vi "HMU Cal - Get Optimal TX IF Frequency.vi"(5 "RF Frequency (Hz)":dbl format="%#_6p", 11 "error in (no error)":errorcluster) -> (6 "IF Frequency (Hz)":dbl format="%#_6p", 15 "error out":errorcluster)   [LabVIEW 2023, in "RFFixtureCharact.RFPM.lvlib" / "SG SC2250 Path.lvclass"]
uses:
  SG SC2250 Path.lvclass
  <vilib>/Utility/error.llb/Error Cluster From Error Code.vi
  <vilib>/ErrorRing/Error Ring.xnode
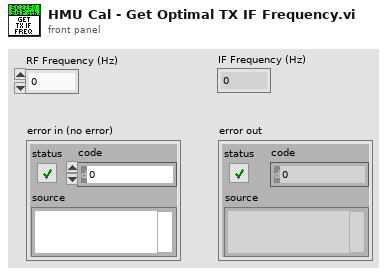
[diagram p1: front panel]
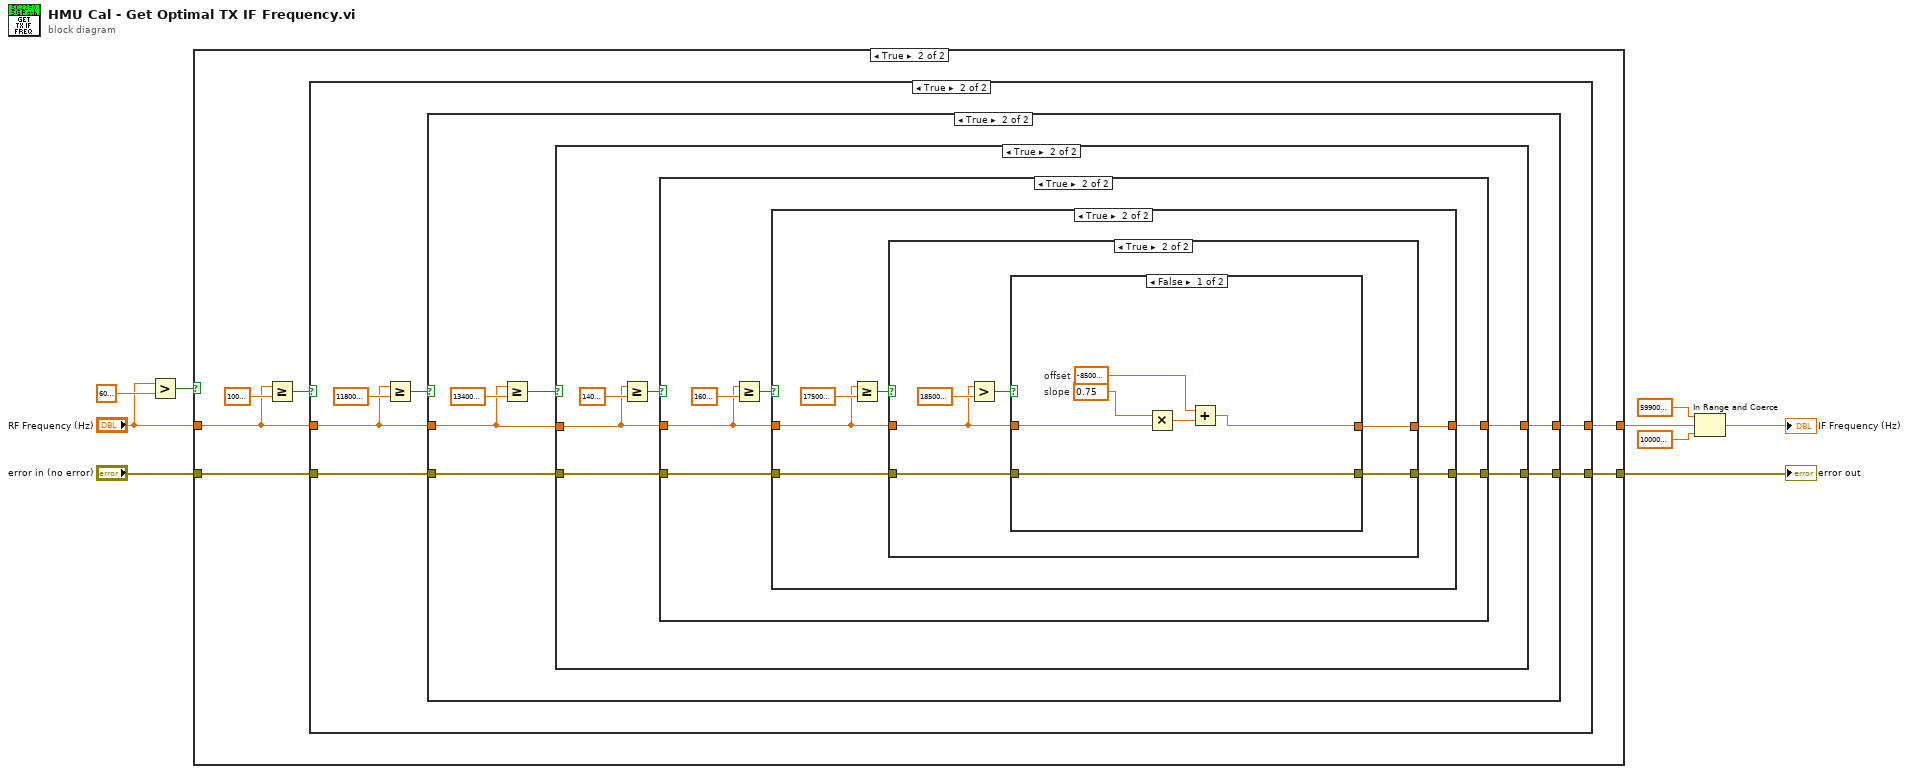
[diagram p0: block diagram]
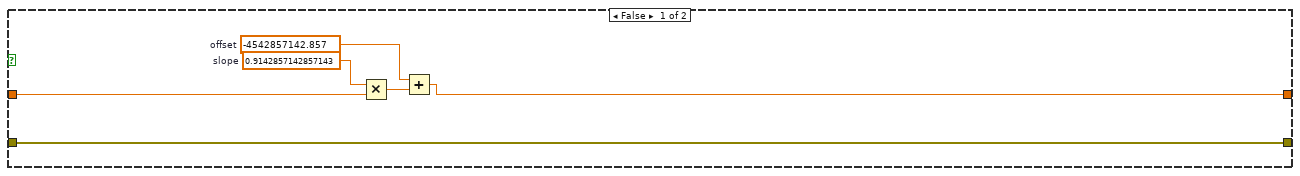
[diagram p3: hidden frame]
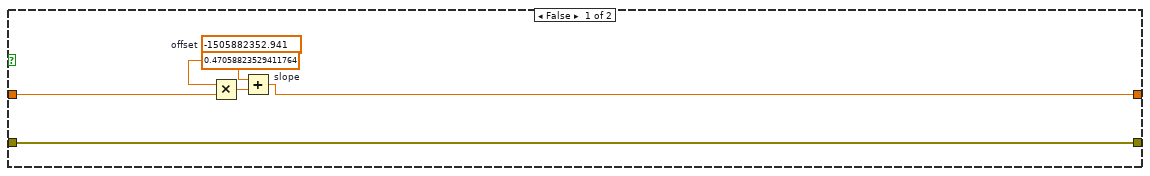
[diagram p4: hidden frame]
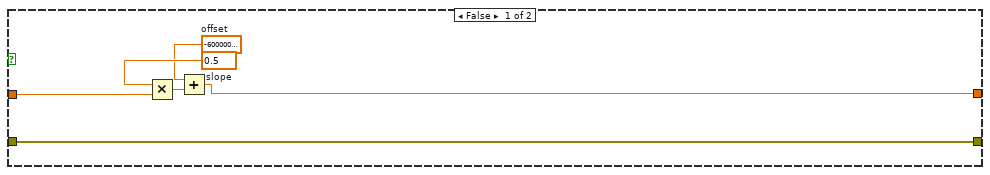
[diagram p5: hidden frame]
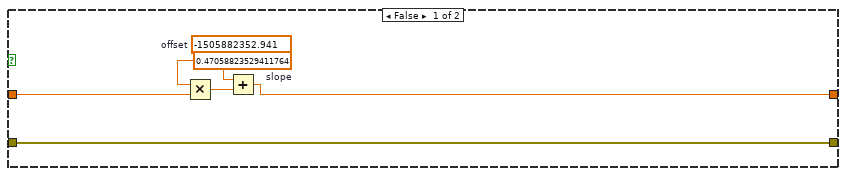
[diagram p6: hidden frame]
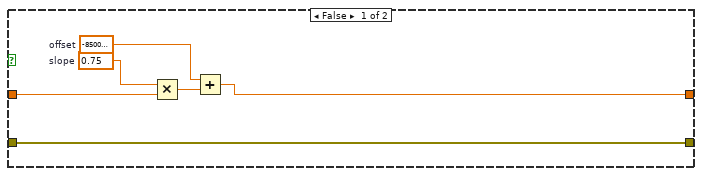
[diagram p7: hidden frame]
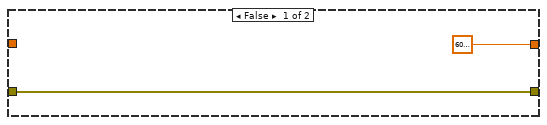
[diagram p8: hidden frame]
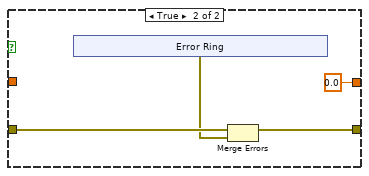
[diagram p9: hidden frame]
diagram:
  n1 = Greater?(x="RF Frequency (Hz)", y=6000000000.0 ("RF Frequency (Hz)")) -> (0:w6:bool)
  n2 = case shown="True" w6 {
    tunnel: "error in (no error)" -> [w11 w12]
    tunnel: [w11 w13] -> w8
    tunnel: "RF Frequency (Hz)" -> [w10 w15]
    tunnel: [w10 w14] -> w4
    frame False {
    }
    frame True {
      n3 = Greater Or Equal?(x=w15, y=10000000000.0 ("RF Frequency (Hz)")) -> (x >= y?=w16:bool)
      n4 = case shown="True" w16 {
        tunnel: w15 -> [w22 w27]
        tunnel: [w19 w26] -> w14
        tunnel: [w18 w25] -> w13
        tunnel: w12 -> [w18 w24]
        frame False {
          w20 = -4542857142.857  # offset
          w21 = 0.9142857142857143  # slope
          n5 = Multiply(x=w21, y=w22) -> (x*y=w23:dbl)
          n6 = Add(x=w20, y=w23) -> (x+y=w19:dbl)
        }
        frame True {
          n7 = Greater Or Equal?(x=w27, y=11800000000.0 ("RF Frequency (Hz)")) -> (x >= y?=w28:bool)
          n8 = case shown="True" w28 {
            tunnel: w27 -> [w32 w37]
            tunnel: [w31 w41] -> w26
            tunnel: [w30 w40] -> w25
            tunnel: w24 -> [w30 w39]
            frame False {
              w33 = -1505882352.941  # offset
              w34 = 0.47058823529411764  # slope
              n9 = Multiply(x=w34, y=w32) -> (x*y=w35:dbl)
              n10 = Add(x=w33, y=w35) -> (x+y=w31:dbl)
            }
            frame True {
              n11 = Greater Or Equal?(x=w37, y=13400000000.0 ("RF Frequency (Hz)")) -> (x >= y?=w36:bool)
              n12 = case shown="True" w36 {
                tunnel: [w43 w51] -> w41
                tunnel: [w42 w50] -> w40
                tunnel: w39 -> [w42 w49]
                tunnel: w37 -> [w44 w48]
                frame False {
                  w45 = -600000000.0  # offset
                  w46 = 0.5  # slope
                  n13 = Multiply(x=w46, y=w44) -> (x*y=w47:dbl)
                  n14 = Add(x=w45, y=w47) -> (x+y=w43:dbl)
                }
                frame True {
                  n15 = Greater Or Equal?(x=w48, y=14000000000.0 ("RF Frequency (Hz)")) -> (x >= y?=w52:bool)
                  n16 = case shown="True" w52 {
                    tunnel: w48 -> [w56 w62]
                    tunnel: [w55 w63] -> w51
                    tunnel: [w54 w61] -> w50
                    tunnel: w49 -> [w54 w60]
                    frame False {
                      w57 = -1505882352.941  # offset
                      w58 = 0.47058823529411764  # slope
                      n17 = Multiply(x=w58, y=w56) -> (x*y=w59:dbl)
                      n18 = Add(x=w57, y=w59) -> (x+y=w55:dbl)
                    }
                    frame True {
                      n19 = Greater Or Equal?(x=w62, y=16000000000.0 ("RF Frequency (Hz)")) -> (x >= y?=w64:bool)
                      n20 = case shown="True" w64 {
                        tunnel: [w67 w72] -> w63
                        tunnel: w62 -> [w68 w73]
                        tunnel: [w66 w76] -> w61
                        tunnel: w60 -> [w66 w77]
                        frame False {
                          w69 = -8500000000.0  # offset
                          w70 = 0.75  # slope
                          n21 = Multiply(x=w70, y=w68) -> (x*y=w71:dbl)
                          n22 = Add(x=w69, y=w71) -> (x+y=w67:dbl)
                        }
                        frame True {
                          n23 = Greater Or Equal?(x=w73, y=17500000000.0 ("RF Frequency (Hz)")) -> (x >= y?=w74:bool)
                          n24 = case shown="True" w74 {
                            tunnel: w77 -> [w78 w85]
                            tunnel: [w78 w84] -> w76
                            tunnel: w73 -> [_ w81]
                            tunnel: [6000000000.0 ("RF Frequency (Hz)") w80] -> w72
                            frame False {
                            }
                            frame True {
                              n25 = Greater?(x=w81, y=18500000000.0 ("RF Frequency (Hz)")) -> (0:w82:bool)
                              n26 = case shown="False" w82 {
                                tunnel: w85 -> [w86 w95]
                                tunnel: [w86 w94] -> w84
                                tunnel: w81 -> [w88 _]
                                tunnel: [w87 0.0 ("RF Frequency (Hz)")] -> w80
                                frame False {
                                w89 = -8500000000.0  # offset
                                w90 = 0.75  # slope
                                n27 = Multiply(x=w90, y=w88) -> (x*y=w91:dbl)
                                n28 = Add(x=w89, y=w91) -> (x+y=w87:dbl)
                                }
                                frame True {
                                n29 = xnode "Error Ring"() -> ("error out"=w93:errorcluster)
                                n30 = Merge Errors(w95, w93) -> (w94:errorcluster)
                                }
                              }
                            }
                          }
                        }
                      }
                    }
                  }
                }
              }
            }
          }
        }
      }
    }
  }
  "error out" <- w8
  n31 = In Range and Coerce(upper limit=5990000000.0 ("RF Frequency (Hz)"), x=w4, lower limit=100000000.0 ("RF Frequency (Hz)")) -> (coerced(x)=→"IF Frequency (Hz)":dbl)  [unwired: 1 out]
